vi "XY Graph Decode Plot Columns Header.vi"(8 "Error In":errorcluster, 9 "Delimiter":string, 10 "Column Header Line? (F)":bool, 11 "Header String Array":string[](array[string])) -> (0 "Error Out":errorcluster, 1 "Plot Scales Array":T1[](array[typedef]), 3 "Plot Name Array":string[](array[string]), 4 "Alternating Axes?":bool)   [LabVIEW 2021, in "XY Graph Add-Ons.lvlib"]
uses:
  XY Graph Add-Ons.lvlib
  XY Graph Plot Scale Labels.ctl
  XY Graph Plot Axis Type.ctl
  Arrays/Signed Array Index.vi
  <vilib>/Utility/error.llb/Error Cluster From Error Code.vi
  <userlib>/_OpenG.lib/array/array.llb/Filter 1D Array with Scalar (I16)__ogtk.vi
  <vilib>/ErrorRing/Error Ring.xnode
  <userlib>/_OpenG.lib/array/array.llb/openg_array.lvlib
  841d8f05-1d7a-43ed-9404-55bcae8d5cf9.vi
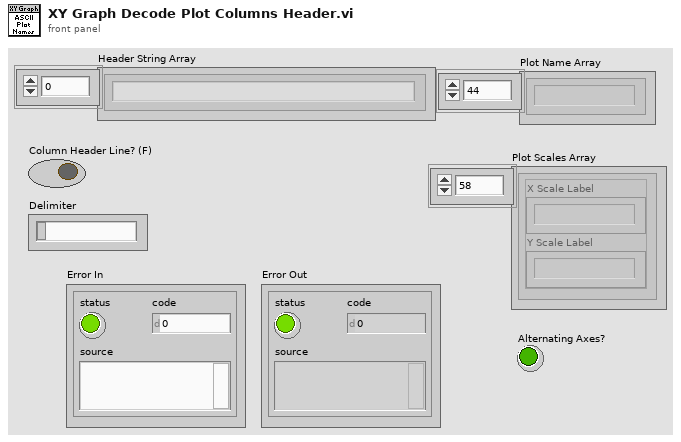
[diagram p1: front panel]
types:
  T1 = typedef "XY Graph Add-Ons.lvlib/XY Graph Plot Scale Labels.ctl" = cluster{"X Scale Label":string, "Y Scale Label":string}
  T2 = typedef "XY Graph Add-Ons.lvlib/XY Graph Plot Axis Type.ctl" = enum16{"X", "Y", "Z", "dX", "dY", "dZ"}
  T3 = cluster{"X Scale Label":string, "Y Scale Label":string}[]
  T4 = cluster{"Scale Label":string, "Scale Label":string}
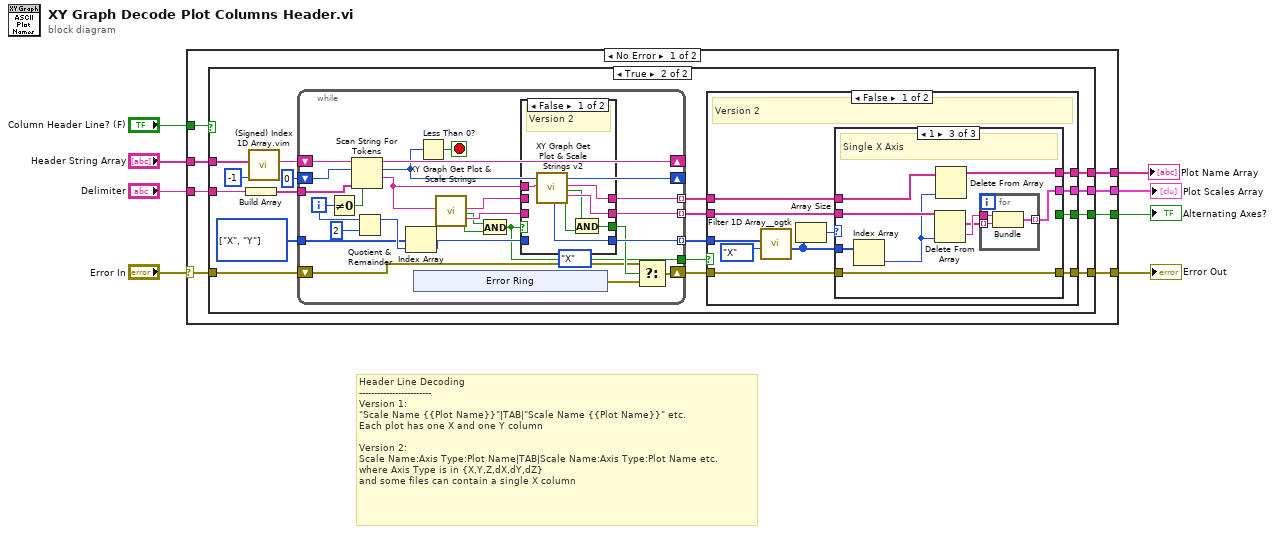
[diagram p0: block diagram]
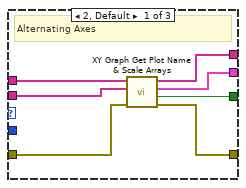
[diagram p3: hidden frame]
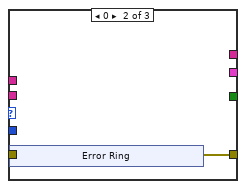
[diagram p4: hidden frame]
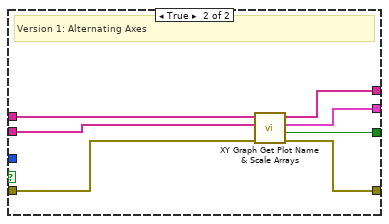
[diagram p5: hidden frame]
diagram:
  # "Header Line Decoding\n------------------------\nVersion 1:\n\"Scale Name {{Plot Name}}\"|TAB|\"Scale Name {{Plot Name}}\" etc.\nEach plot has one X and one Y column\n\nVersion 2:\nScale Name:Axis Type:Plot Name|TAB|Scale Name:Axis Type:Plot Name etc.\nwhere Axis Type is in {X,Y,Z,dX,dY,dZ}\nand some files can contain a single X column"
  n1 = case shown="No Error" "Error In" {
    selector: "Error In" -> [w10 w117]
    tunnel: "Delimiter" -> [w16 _]
    tunnel: "Header String Array" -> [w15 _]
    tunnel: "Column Header Line? (F)" -> [w14 _]
    tunnel: [w13 _] -> w1
    tunnel: [w12 _] -> w2
    tunnel: [w11 _] -> w3
    tunnel: [w9 w117] -> w4
    frame No Error {
      n2 = case shown="True" w14 {
        tunnel: w15 -> [_ w34]
        tunnel: w16 -> [_ w31]
        tunnel: [_ w27] -> w13
        tunnel: [_ w25] -> w12
        tunnel: [_ w24] -> w11
        tunnel: w10 -> [w17 w22]
        tunnel: [w17 w19] -> w9
        frame False {
        }
        frame True {
          w23 = T2[] [enum."X", enum."Y"] items=["X", "Y", "Z", "dX", "dY", "dZ"] ("Array")
          n3 = Build Array(w31) -> (w30:string[])
          n4 = call "(Signed) Index 1D Array.vim"("Signed Index"=-1, "Array"=w34) -> ("Array Element"=w32:string)  [unwired: 9 in]
          n5 = while {
            shift-right: [w100] -> _
            shift-left: w32 -> [w101]
            shift-right: [w96] -> _
            shift-left: 0 ("offset past token") -> [w99]
            tunnel: w30 -> [w98]
            tunnel: [w93] -> w26 mode=indexing
            tunnel: [w94] -> w28 mode=indexing
            tunnel: [w92] -> w18 mode=indexing
            tunnel: w23 -> [w88]
            shift-right: [w84] -> w20
            shift-left: w22 -> [w85]
            tunnel: [w83] -> w21
            i -> [w91]
            stop <- w95 stop-if-true
            n6 = Not Equal To 0?(x=w91) -> (x != 0?=w97:bool)
            n7 = Scan String For Tokens(4:w97, 6:w98, 8:w99, 9:w101) -> (1:w81:string, 2:w96:i32, 3:w100:string)  [unwired: 2 in, 1 out]
            n8 = Quotient & Remainder(x=w91, y=2) -> (x-y*floor(x/y)=w89:i32)  [unwired: 1 out]
            n9 = Index Array(array=w88, index=w89) -> (element=w87:T2)
            n10 = xnode "Error Ring"() -> ("error out"=w82:errorcluster)
            n11 = Less Than 0?(x=w96) -> (x < 0?=w95:bool)
            n12 = call "XY Graph Get Plot & Scale Strings.vi"("Plot Column Header"=w81) -> ("Plot Name"=w80:string, "Valid Plot Name?"=w77:bool, "Scale Label"=w78:string, "Valid Scale Name?"=w79:bool)  [unwired: 15 in]
            n13 = And(x=w77, y=w79) -> (x .and. y?=w83:bool)
            n14 = case shown="False" w83 {
              selector: w83 -> [_ w113]
              tunnel: w80 -> [_ w116]
              tunnel: w78 -> [_ w115]
              tunnel: [w109 w116] -> w94
              tunnel: [w108 w115] -> w93
              tunnel: w81 -> [w112 _]
              tunnel: [w111 w114] -> w92
              tunnel: w87 -> [_ w114]
              tunnel: [w110 w113] -> w86
              frame False {
                (unwired) XY_Graph_Plot_Axis_Type."X" ("Axis Type")
                # "Version 2"
                n15 = call "XY Graph Get Plot & Scale Strings v2.vi"("Plot Column Header"=w112) -> ("Axis Type"=w111:T2, "Plot Name"=w109:string, "Valid Plot Name?"=w107:bool, "Scale Label"=w108:string, "Valid Scale Name?"=w106:bool)  [unwired: 14 in]
                n16 = And(x=w107, y=w106) -> (x .and. y?=w110:bool)
              }
              frame True {
                # "X, Y alternate"
                # "Version 1"
              }
            }
            n17 = Select(t=w85, s=w86, f=w82) -> (s? t:f=w84:errorcluster)
          }
          n18 = case shown="False" w21 {
            tunnel: w28 -> [w42 w76]
            tunnel: [w39 w75] -> w27
            tunnel: w26 -> [w41 w74]
            tunnel: [w36 w70] -> w25
            tunnel: [w37 w73] -> w24
            tunnel: w20 -> [w35 w71]
            tunnel: [w38 w72] -> w19
            tunnel: w18 -> [w45 _]
            frame False {
              # "Version 2"
              n19 = call-poly <userlib>:"Filter 1D Array__ogtk.vi"("items to filter"=XY_Graph_Plot_Axis_Type."X" ("Axis Type"), "array"=w45) -> ("filtered item indices"=w40:i32[])  [unwired: 4 in, 1 out]
              n20 = Array Size(array=w40) -> (size(s)=w43:i32)
              n21 = case shown="1" w43 {
                tunnel: w42 -> [w52 _ w62]
                tunnel: w41 -> [w51 _ w65]
                tunnel: w40 -> [_ _ w66]
                tunnel: [w50 _ w60] -> w39
                tunnel: [w48 w53 w58] -> w38
                tunnel: [w49 _ w59] -> w37
                tunnel: [w47 _ _] -> w36
                tunnel: w35 -> [w46 _ w58]
                frame 2, Default {
                  # "Alternating Axes"
                  n22 = call "XY Graph Get Plot Name & Scale Arrays.vi"("error in"=w46, "Scale Labels in"=w51, "Plot Names in"=w52) -> ("error out"=w48:errorcluster, "Alternating Axes?"=w47:bool, "Plot Scales Array"=w49:T3, "Plot Names Array"=w50:string[])  [unwired: 5 in]
                }
                frame 0 {
                  n23 = xnode "Error Ring"() -> ("error out"=w53:errorcluster)
                }
                frame 1 {
                  # "Single X Axis"
                  n24 = Index Array(array=w66) -> (element=w61:i32)  [unwired: 1 in]
                  n25 = Delete From Array(array=w65, index=w61) -> (deleted portion=w64:string, array with subset deleted=w63:string[])  [unwired: 1 in]
                  n26 = Delete From Array(array=w62, index=w61) -> (array with subset deleted=w60:string[])  [unwired: 1 in, 1 out]
                  n27 = for {
                    tunnel: w64 -> [w69]
                    tunnel: w63 -> [w68] mode=indexing
                    tunnel: [w67] -> w59 mode=indexing
                    n28 = Bundle("Scale Label"=w69, "Scale Label"=w68) -> (w67:T4)  [unwired: 1 in]
                  }
                }
              }
            }
            frame True {
              # "Version 1: Alternating Axes"
              n29 = call "XY Graph Get Plot Name & Scale Arrays.vi"("error in"=w71, "Scale Labels in"=w74, "Plot Names in"=w76) -> ("error out"=w72:errorcluster, "Alternating Axes?"=w70:bool, "Plot Scales Array"=w73:T3, "Plot Names Array"=w75:string[])  [unwired: 5 in]
            }
          }
        }
      }
    }
    frame Error {
    }
  }
  "Plot Name Array" <- w1
  "Error Out" <- w4
  "Plot Scales Array" <- w3
  "Alternating Axes?" <- w2
